vi "Serial Transmit Receive Simulation.vi"() -> ()   [LabVIEW 2013]
uses:
  <vilib>/rvi/DesktopExecutionNode/Execution/niFpgaDEN_Execute.vi
  <vilib>/rvi/DesktopExecutionNode/DesktopExecutionNode.xnode
  Source/I2S-TDM.lvlib
panel:
  out "sample out bits":bool[](array[boolean])
  in  "force stop":bool
  in  "ready for output":bool
  out "sample in":u32
  out "sample out":u32
  in  "start transfer":bool
  in  "pause":bool
  in  "24-bit data":bool[](array[boolean])=[TRUE, FALSE, FALSE, FALSE, FALSE, FALSE, FALSE, FALSE, FALSE, FALSE, FALSE, FALSE, FALSE, FALSE, FALSE, FALSE, FALSE, FALSE, FALSE, FALSE, FALSE, FALSE, FALSE, TRUE]
  in  "wait":u32=50
  out "Digital Waveform Graph":digitalwaveform(graph)
  in  "input valid":bool
  in  "transfer length":u8=32
  in  "stop":bool
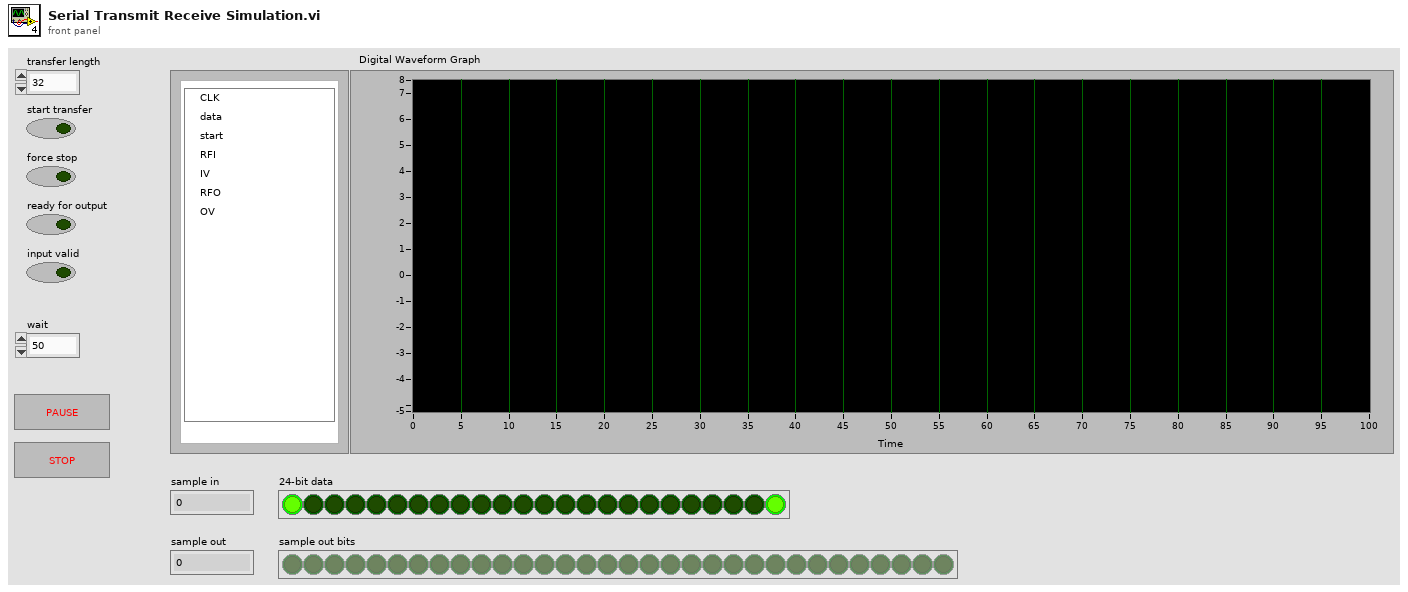
[diagram p1: front panel]
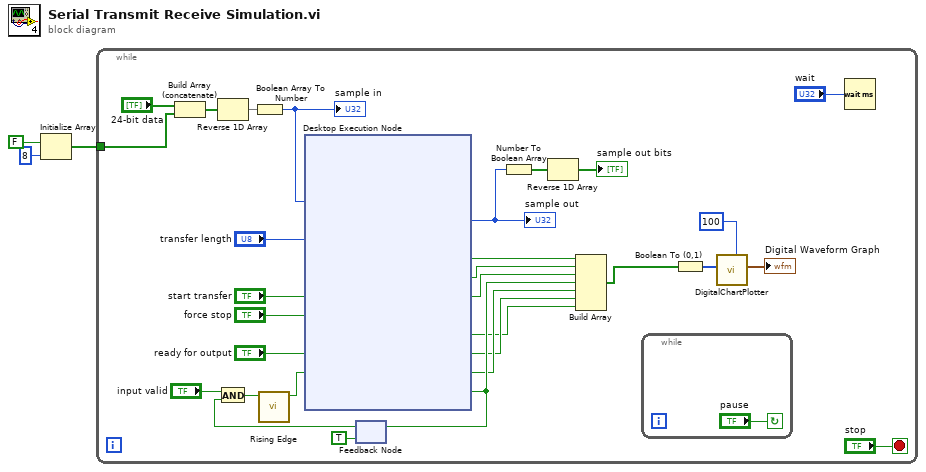
[diagram p0: block diagram]
diagram:
  n1 = Initialize Array(FALSE, 8 ("dimension size")) -> (w1:bool[])
  n2 = while {
    tunnel: w1 -> [w28]
    stop <- "stop" stop-if-true
    n3 = Build Array (concatenate)("24-bit data", w28) -> (w27:bool[])
    n4 = Reverse 1D Array(array=w27) -> (reversed array=w26:bool[])
    n5 = Boolean Array To Number(Boolean array=w26) -> (number=w22:u32)
    "sample in" <- w22
    n6 = feedback #1(TRUE ("ready for input")) -> (w18:bool)
    n7 = And(x="input valid", y=w18) -> (x .and. y?=w20:bool)
    n8 = call "Rising Edge.vi"("signal in"=w20) -> ("rising edge?"=w19:bool)  [unwired: 10 in]
    n9 = xnode "Desktop Execution Node"("sample in"=w22, "transfer length"="transfer length", "start transfer"="start transfer", "force stop"="force stop", "ready for output"="ready for output", "input valid"=w19) -> ("sample out"=w8:u32, "clk"=w24:bool, "data"=w4:bool, "start transfer"=w5:bool, "output valid"=w12:bool, "ready for output"=w13:bool, "input valid"=w14:bool, "ready for input"=w15:bool)  [unwired: 1 in, 1 out]
    "sample out" <- w8
    n10 = feedback-in #1(w15) -> ()
    n11 = Number To Boolean Array(number=w8) -> (Boolean array=w7:bool[])
    n12 = Reverse 1D Array(array=w7) -> (reversed array=→"sample out bits":bool[])
    n13 = Build Array(w24, w4, w5, w15, w14, w13, w12) -> (w11:bool[])
    n14 = while {
      stop <- "pause" continue-if-true
    }
    n15 = Boolean To (0,1)(Boolean=w11) -> (0, 1=w10:i16[])
    n16 = call "DigitalChartPlotter.vi"("History Size"=100, "Input"=w10) -> ("Digital Data"=→"Digital Waveform Graph":digitalwaveform)  [unwired: 9 in]
    n17 = Wait (ms)(milliseconds to wait="wait") -> ()  [unwired: 1 out]
  }
